vi "Read NumberOfRobots.vi"(8 "error in (no error)":errorcluster, 11 "BallPlacementAllyPlay in":refnum<class "BallPlacementAllyPlay.lvclass">) -> (0 "error out":errorcluster, 2 "NumberOfRobots":u32=6, 3 "BallPlacementAllyPlay out":refnum<class "BallPlacementAllyPlay.lvclass">)   [LabVIEW 2021, in "BallPlacementAllyPlay.lvclass"]
uses:
  BallPlacementAllyPlay.lvclass
  BallPlacementAllyPlay.lvclass/BallPlacementAllyPlay.ctl
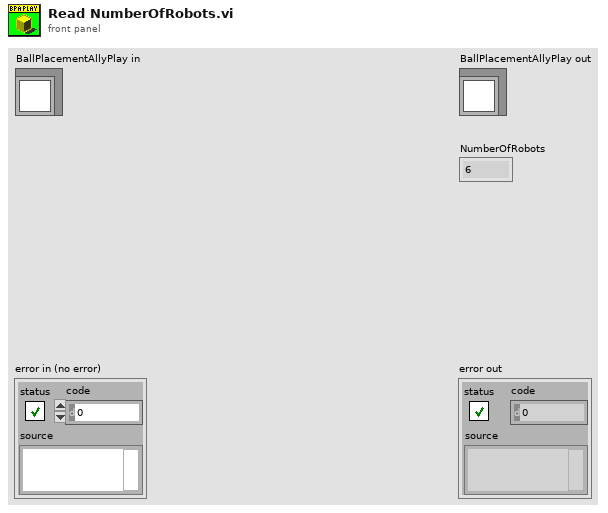
[diagram p1: front panel]
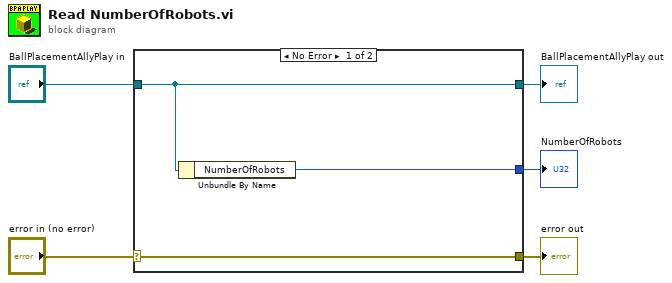
[diagram p0: block diagram]
diagram:
  n1 = case shown="No Error" "error in (no error)" {
    selector: "error in (no error)" -> [w8 w9]
    tunnel: [w8 w9] -> w4
    tunnel: [w7 w10] -> w2
    tunnel: "BallPlacementAllyPlay in" -> [w7 w10]
    tunnel: [w6 _] -> w1
    frame No Error {
      n2 = Unbundle By Name(w7) -> ("NumberOfRobots"=w6:u32)
    }
    frame Error {
    }
  }
  "error out" <- w4
  "BallPlacementAllyPlay out" <- w2
  "NumberOfRobots" <- w1
